vi "getFilter.vi"(8 "error in (no error)":errorcluster, 11 "ZTAAC in":refnum<class "ZTAAC.lvclass">) -> (0 "error out":errorcluster, 2 "Filter Type":T1, 3 "ZTAAC out":refnum<class "ZTAAC.lvclass">)   [LabVIEW 2016, in "OfcFunc.lvlib" / "ZTAAC.lvclass"]
doc: "Get the active filter type."
uses:
  ZTAAC.lvclass
  StrictDef/FilterType.ctl
  ZTAAC.lvclass/ZTAAC.ctl
  OfcFunc.lvlib
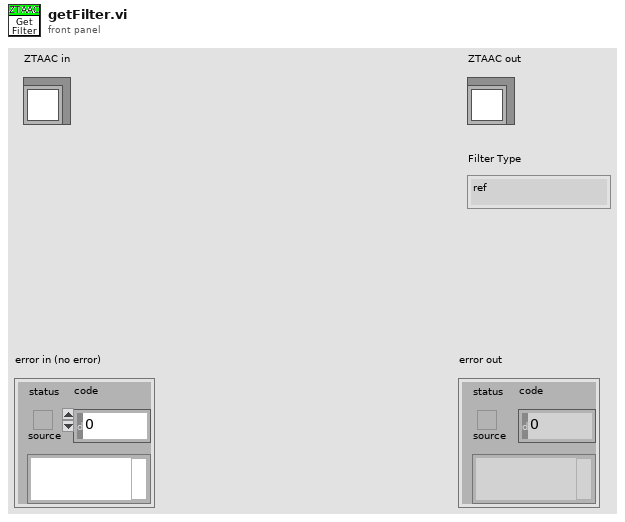
[diagram p1: front panel]
types:
  T1 = typedef "OfcFunc.lvlib/FilterType.ctl" = enum16{"ref", "u", "g", "r", "i", "z", "y"}
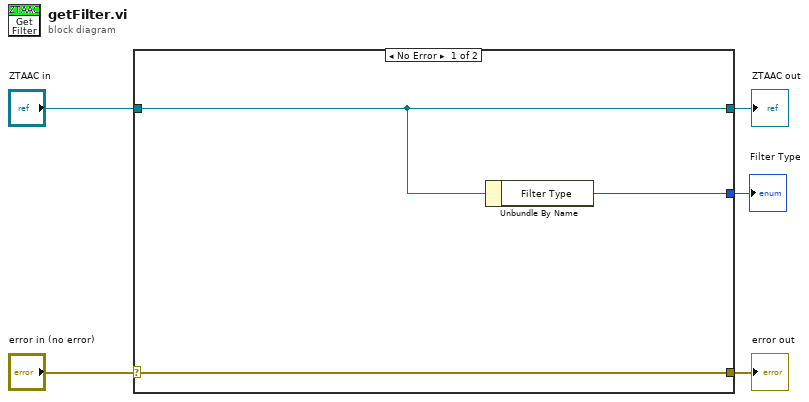
[diagram p0: block diagram]
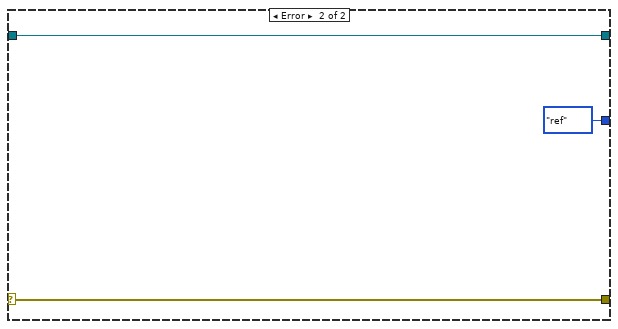
[diagram p2: hidden frame]
diagram:
  n1 = case shown="No Error" "error in (no error)" {
    selector: "error in (no error)" -> [w8 w11]
    tunnel: [w8 w11] -> w4
    tunnel: [w7 w10] -> w2
    tunnel: "ZTAAC in" -> [w7 w10]
    tunnel: [w6 FilterType."ref" ("Filter Type")] -> w1
    frame No Error {
      n2 = Unbundle By Name(w7) -> ("Filter Type"=w6:T1)
    }
    frame Error {
    }
  }
  "error out" <- w4
  "ZTAAC out" <- w2
  "Filter Type" <- w1
